vi "Write Metrics.vi"(8 "error in (no error)":errorcluster, 10 "Metrics":map{string, refnum<data-value>}(c390), 11 "Registry Session in":refnum<class "Registry Session.lvclass">) -> (0 "error out":errorcluster, 3 "Registry Session out":refnum<class "Registry Session.lvclass">)   [LabVIEW 2020, in "Registry.lvlib" / "Registry Session.lvclass"]
uses:
  Registry Session.lvclass
  metrics/metric/Metric.lvclass
  Registry Session.lvclass/Registry Session.ctl
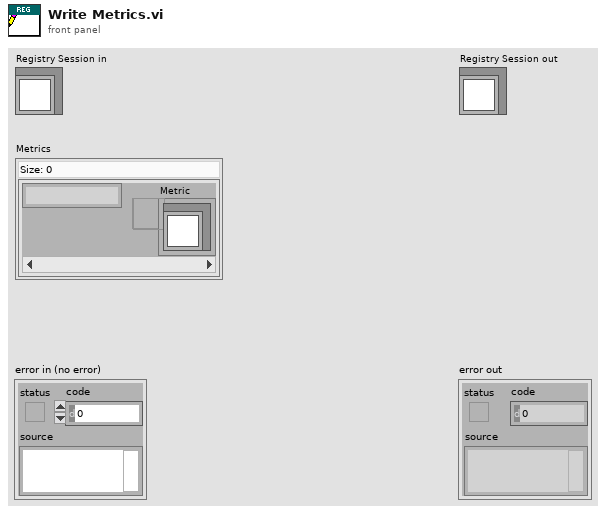
[diagram p1: front panel]
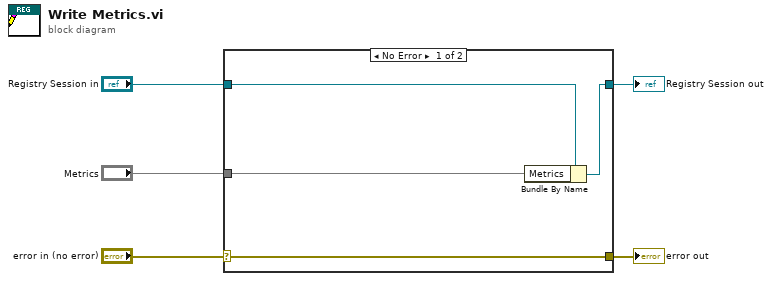
[diagram p0: block diagram]
diagram:
  n1 = case shown="No Error" "error in (no error)" {
    selector: "error in (no error)" -> [w9 w10]
    tunnel: [w9 w10] -> w4
    tunnel: [w7 w11] -> w2
    tunnel: "Registry Session in" -> [w8 w11]
    tunnel: "Metrics" -> [w6 _]
    frame No Error {
      n2 = Bundle By Name(cluster=w8, "Metrics"=w6) -> (w7:refnum<class "Registry Session.lvclass">)
    }
    frame Error {
    }
  }
  "error out" <- w4
  "Registry Session out" <- w2
